vi "Get Image.vi"(8 "error in":errorcluster, 9 "Image In":T1, 10 "Camera Name":string, 11 "Gantry in":refnum<class "Gantry Class.lvclass">) -> (0 "error out":errorcluster, 2 "Image Out":T1, 3 "Gantry out":refnum<class "Gantry Class.lvclass">)   [LabVIEW 2011, in "Gantry Class.lvclass"]
uses:
  Gantry Class.lvclass
  <vilib>/vision/Image Controls.llb/IMAQ Image.ctl
  <vilib>/vision/driver/NI_Vision_Acquisition_Software.lvlib
  <vilib>/vision/NI_Vision_Development_Module.lvlib
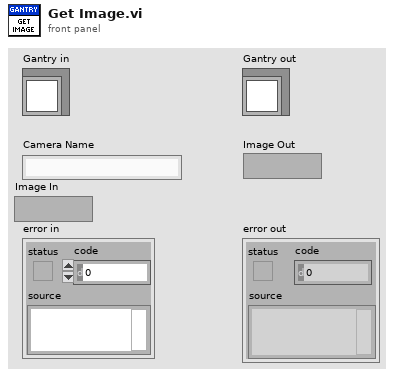
[diagram p1: front panel]
types:
  T1 = typedef "IMAQ Image.ctl" = refnum<image>
  T2 = typedef "Image Type" = u32
  T3 = typedef "Gantry_Camera.ctl" = cluster{"Name":string, "IMAQ Session":T4, "Group":u32, "Open?":bool, "Interface Name":string}
  T4 = typedef "IMAQdx.ctl" = refnum<k21>
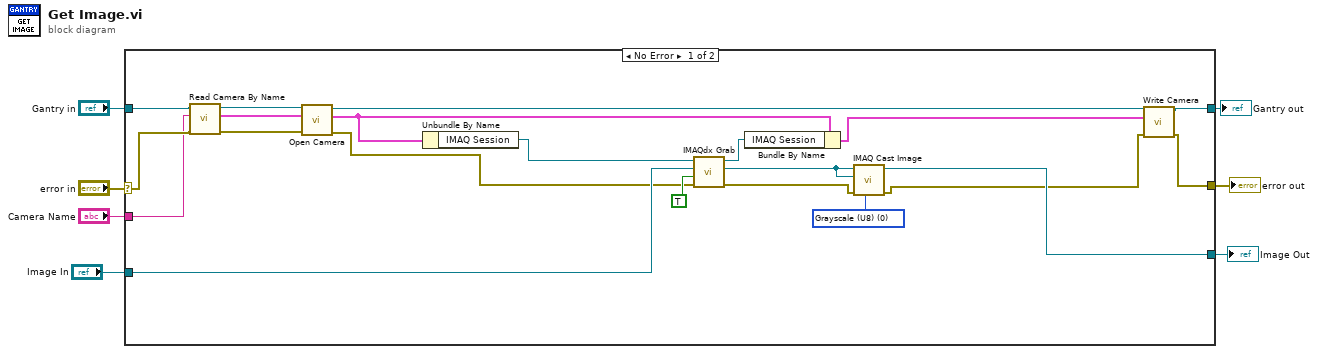
[diagram p0: block diagram]
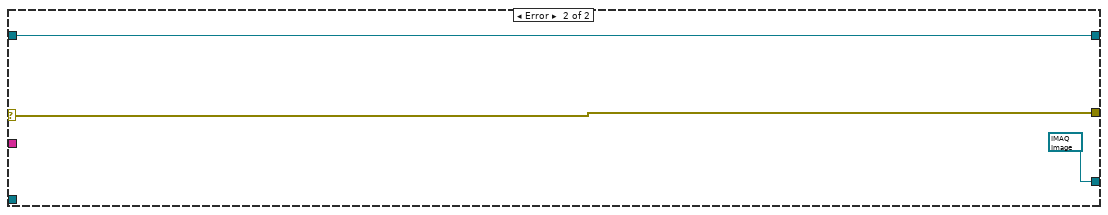
[diagram p2: hidden frame]
diagram:
  n1 = case shown="No Error" "error in" {
    selector: "error in" -> [w24 w31]
    tunnel: [w25 w31] -> w6
    tunnel: [w26 w30] -> w4
    tunnel: "Gantry in" -> [w27 w30]
    tunnel: [w20 T1 refnum ("Image Out")] -> w3
    tunnel: "Camera Name" -> [w10 _]
    tunnel: "Image In" -> [w9 _]
    frame No Error {
      w21 = T2 0 items=["Grayscale (U8)", "Grayscale (I16)", "Grayscale (SGL)", "Complex (CSG)", "RGB (U32)", "HSL (U32)", "RGB (U64)", "Grayscale (U16)"] ("Image Type")
      n2 = call-dynamic "Read Camera By Name.vi"("error in (no error)"=w24, "Camera Name"=w10, "Gantry Class in"=w27) -> ("error out"=w15:errorcluster, "Camera"=w16:T3, "Gantry Class out"=w17:refnum<class "Gantry Class.lvclass">)  [unwired: 6 in]
      n3 = call-dynamic "Open Camera.vi"("error in (no error)"=w15, "Camera"=w16, "Gantry Class in"=w17) -> ("error out"=w8:errorcluster, "Camera Out"=w14:T3, "Gantry Class out"=w13:refnum<class "Gantry Class.lvclass">)  [unwired: 6 in]
      n4 = Unbundle By Name(w14) -> ("IMAQ Session"=w19:T4)
      n5 = call <vilib>:"IMAQdx Grab.vi"("error in"=w8, "Wait for Next Buffer? (Yes)"=TRUE, "Image In"=w9, "Session In"=w19) -> ("error out"=w18:errorcluster, "Image Out"=w12:T1, "Session Out"=w28:T4)  [unwired: 4 in, 1 out]
      n6 = Bundle By Name(cluster=w14, "IMAQ Session"=w28) -> (w23:T3)
      n7 = call "IMAQ Cast Image"("Image Type"=w21, "error in (no error)"=w18, "Image Dst"=w12, "Image Src"=w12) -> ("error out"=w11:errorcluster, "Image Dst Out"=w20:T1)  [unwired: 6 in]
      n8 = call-dynamic "Write Camera.vi"("error in (no error)"=w11, "Camera"=w23, "Gantry Class in"=w13) -> ("error out"=w25:errorcluster, "Gantry Class out"=w26:refnum<class "Gantry Class.lvclass">)  [unwired: 6 in]
    }
    frame Error {
    }
  }
  "error out" <- w6
  "Gantry out" <- w4
  "Image Out" <- w3
